vi "Read Base.vi"(8 "error in (no error)":errorcluster, 11 "Base Class Test In":refnum<class "Base Test.lvclass">) -> (0 "error out":errorcluster, 2 "Base.lvclass":refnum<class "Base.lvclass">, 3 "Base Class Test Out":refnum<class "Base Test.lvclass">)   [LabVIEW 2020, in "Base Test.lvclass"]
uses:
  Base Test.lvclass
  Framework/Base/Base.lvclass
  Base Test.lvclass/Base Test.ctl
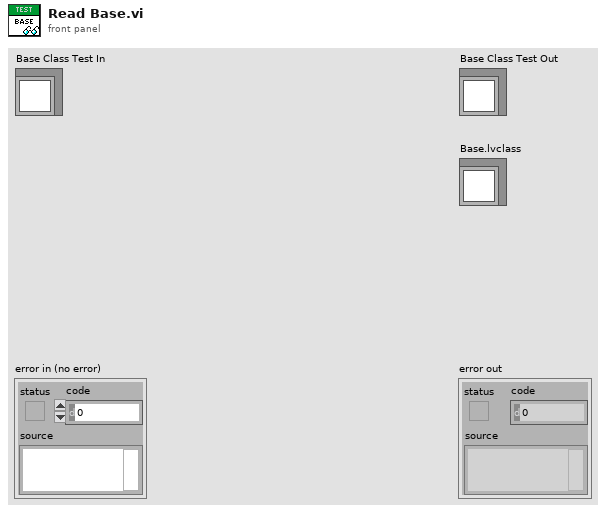
[diagram p1: front panel]
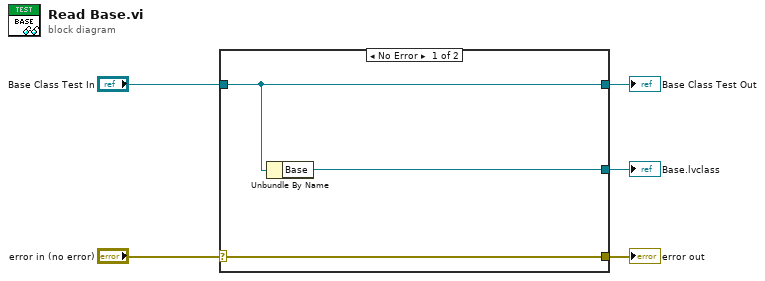
[diagram p0: block diagram]
diagram:
  n1 = case shown="No Error" "error in (no error)" {
    selector: "error in (no error)" -> [w8 w9]
    tunnel: [w8 w9] -> w4
    tunnel: [w7 w10] -> w2
    tunnel: "Base Class Test In" -> [w7 w10]
    tunnel: [w6 _] -> w1
    frame No Error {
      n2 = Unbundle By Name(w7) -> ("Base"=w6:refnum<class "Base.lvclass">)
    }
    frame Error {
    }
  }
  "error out" <- w4
  "Base Class Test Out" <- w2
  "Base.lvclass" <- w1
